vi "setFgenFreqWait.vi"(8 "error in (no error)":errorcluster, 9 "Frequency":dbl, 10 "Channel":string, 11 "Instrument handle":refnum<k15>) -> (0 "error out":errorcluster, 3 "Instrument handle out":refnum<k15>)   [LabVIEW 2020]
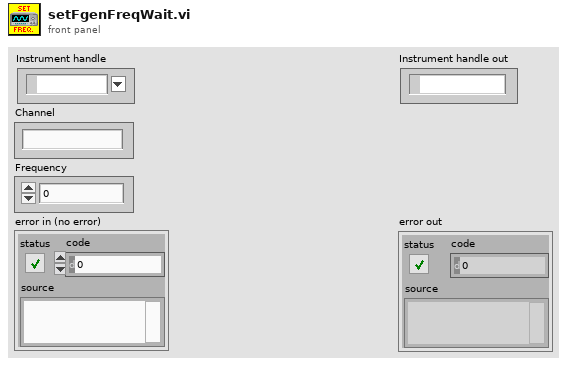
[diagram p1: front panel]
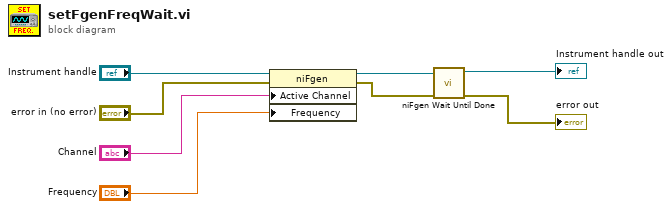
[diagram p0: block diagram]
diagram:
  n1 = property class="niFgen"(reference="Instrument handle", error in="error in (no error)", "Active Channel"="Channel", "Frequency"="Frequency") -> (reference out=w4:refnum<k15>, error out=w3:errorcluster)
  n2 = call <instrlib>:"niFgen Wait Until Done.vi"("error in (no error)"=w3, "Instrument Handle"=w4) -> ("error out"=→"error out":errorcluster, "Instrument Handle Out"=→"Instrument handle out":refnum<k15>)  [unwired: 8 in]
